vi "Autonomous Independent.vi"   [LabVIEW 2016]
doc: "This VI is called when autonomous begins, and will automatically be terminated when autonomous ends. You can carry out timed or sensor driven robot movement independently without needing to return to the caller."
uses:
  <vilib>/Rock Robotics/WPI/Utilities/WPI_GetSetVariantRefNum.vi
  Accordian/placed.vi
  External/Auto.vi
types:
  T1 = typedef "WPI_RobotDriveDevRef.ctl" = cluster{"DevStatus":errorcluster, "Motors[]":T2[], "Square Inputs":bool, "Max Output":dbl}
  T2 = typedef "WPI_MotorControlDeviceRef.ctl" = cluster{"DeviceStatus":errorcluster, "Type":T3, "PWM":cluster{"PWM Channel":T4, "DeadBand":T5}, "CAN":cluster{"Device Number":u8, "SetOutput VI Ref":variant, "GetOutput VI Ref":variant, "Enable VI Ref":variant, "Disable VI Ref":variant, "Data":variant}, "Invert":bool}
  T3 = typedef "WPI_MotorControlType.ctl" = enum16{"PWM", "CAN"}
  T4 = typedef "FPGA_DIOPWMChannel.ctl" = enum8{"PWM 0", "PWM 1", "PWM 2", "PWM 3", "PWM 4", "PWM 5", "PWM 6", "PWM 7", "PWM 8", "PWM 9", "PWM MXP 0", "PWM MXP 1", "PWM MXP 2", "PWM MXP 3", "PWM MXP 4", "PWM MXP 5", "PWM MXP 6", "PWM MXP 7", "PWM MXP 8", "PWM MXP 9", "Invalid"}
  T5 = typedef "WPI_PWMDeadband.ctl" = cluster{"Name":string, "maxPositivePwm":i32, "minPositivePwm":i32, "centerPwm":i32, "maxNegativePwm":i32, "minNegativePwm":i32, "angularRange":u16}
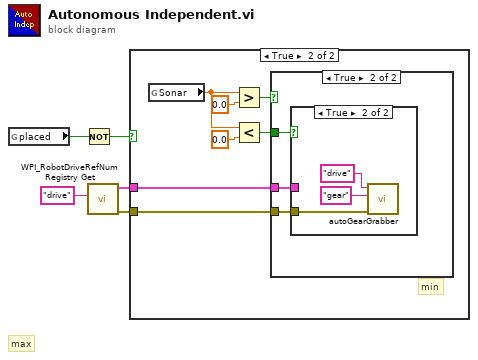
[diagram p0: block diagram]
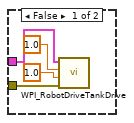
[diagram p3: hidden frame]
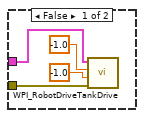
[diagram p4: hidden frame]
diagram:
  # "max"
  n1 = global read "placed.vi" "placed"() -> (w5:bool)
  n2 = Not(x=w5) -> (.not. x?=w4:bool)
  n3 = call <vilib>:"WPI_RobotDriveRefNum Registry Get.vi"("refnum name"="drive") -> ("error out"=w1:errorcluster, "RobotDriveDevRef"=w2:T1)  [unwired: 9 in]
  n4 = case shown="True" w4 {
    tunnel: w2 -> [_ w9]
    tunnel: w1 -> [_ w8]
    frame False {
    }
    frame True {
      # "min"
      n5 = global read "Auto.vi" "Sonar"() -> (w12:dbl)
      n6 = Greater?(x=w12, y=0.0) -> (0:w7:bool)
      n7 = Less?(x=w12, y=0.0) -> (x < y?=w6:bool)
      n8 = case shown="True" w7 {
        tunnel: w9 -> [w14 w17]
        tunnel: w8 -> [w13 w18]
        tunnel: w6 -> [_ w19]
        frame False {
          n9 = call <vilib>:"WPI_RobotDriveTankDrive.vi"("error in (no error)"=w13, "Right axis value"=1.0, "Left axis value"=1.0, "RobotDriveDevRef"=w14) -> ()  [unwired: 5 in, 3 out]
        }
        frame True {
          n10 = case shown="True" w19 {
            tunnel: w18 -> [w21 w24]
            tunnel: w17 -> [w20 _]
            frame False {
              n11 = call <vilib>:"WPI_RobotDriveTankDrive.vi"("error in (no error)"=w21, "Right axis value"=-1.0, "Left axis value"=-1.0, "RobotDriveDevRef"=w20) -> ()  [unwired: 5 in, 3 out]
            }
            frame True {
              n12 = call "autoGearGrabber.vi"("error in (no error)"=w24, "gear"="gear", "drive"="drive") -> ()  [unwired: 8 in, 1 out]
            }
          }
        }
      }
    }
  }
